vi "Close1.vi"(8 "error in (no error)":errorcluster, 11 "VISA resource name":refnum<visa-resource-name>) -> (0 "error out":errorcluster)   [LabVIEW 2015, in "Agilent 3446X Series1.lvlib"]
doc: "Performs an instrument error query before terminating the software connection to the instrument."
uses:
  Agilent 3446X Series1.lvlib
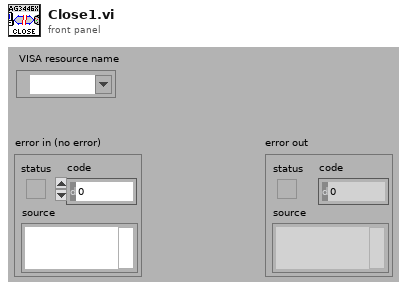
[diagram p1: front panel]
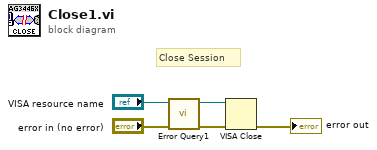
[diagram p0: block diagram]
diagram:
  # "Close Session"
  n1 = call "Error Query1.vi"("error in (no error)"="error in (no error)", "VISA resource name"="VISA resource name") -> ("error out"=w2:errorcluster, "VISA resource name out"=w1:refnum<visa-resource-name>)  [unwired: 8 out]
  n2 = VISA Close(VISA resource name=w1, error in (no error)=w2) -> (error out=→"error out":errorcluster)
